vi "send_solutionChange-v01.vi"(0 "daq_ao 2":tag="Dev1/ao1", 1 "Duration (s)":dbl, 2 "controls array in":refnum<vi>[](array[refnum]), 3 "Sample Freq (Hz)":dbl min=0.0 max=40000.0, 4 "Phase":dbl, 5 "Duty Cycle":dbl, 6 "daq_ai":tag="Dev1/ai0:1", 8 "daq_do":tag="Dev1/ai0:1", 9 "Number of Replicates":i16=1 min=1 max=10, 10 "Start Position":T1(ring), 11 "common cluster":T2, 12 "Jump Position":T1(ring), 13 "error in":errorcluster) -> (14 "output cluster":T3={"daq_ao"="", "Duration (s)"=0.0, "Sample Freq (Hz)"=0.0, "Phase"=0.0, "Duty Cycle"=0.0, "Number of Replicates"=1} {"Number of Replicates" min=1 max=10}, 15 "output waveform":waveform(dbl), 16 "control array out":refnum<vi>[](array[refnum]), 18 "error out":errorcluster, 19 "jumptestMonitor":waveform(dbl)[](graph))   [LabVIEW 2019]
uses:
  multipatch/controls/multipatch_common_controls_v4.ctl
  machine_vision/controls/transform_cluster_actuator.ctl
  machine_vision/coordinate model vis/transform_properties_actuators.ctl
  pipette cleaning/pressure box/cleaning_soft/controls/actuator_cluster.ctl
  pipette cleaning/pressure box/cleaning_soft/controls/actuator_type.ctl
  pipette cleaning/pressure box/cleaning_soft/controls/pressure_box_control.ctl
  pipette cleaning/pressure box/cleaning_soft/controls/pressure_box_type.ctl
  controls/NH_method.ctl
  <vilib>/measure/NI_MABase.lvlib
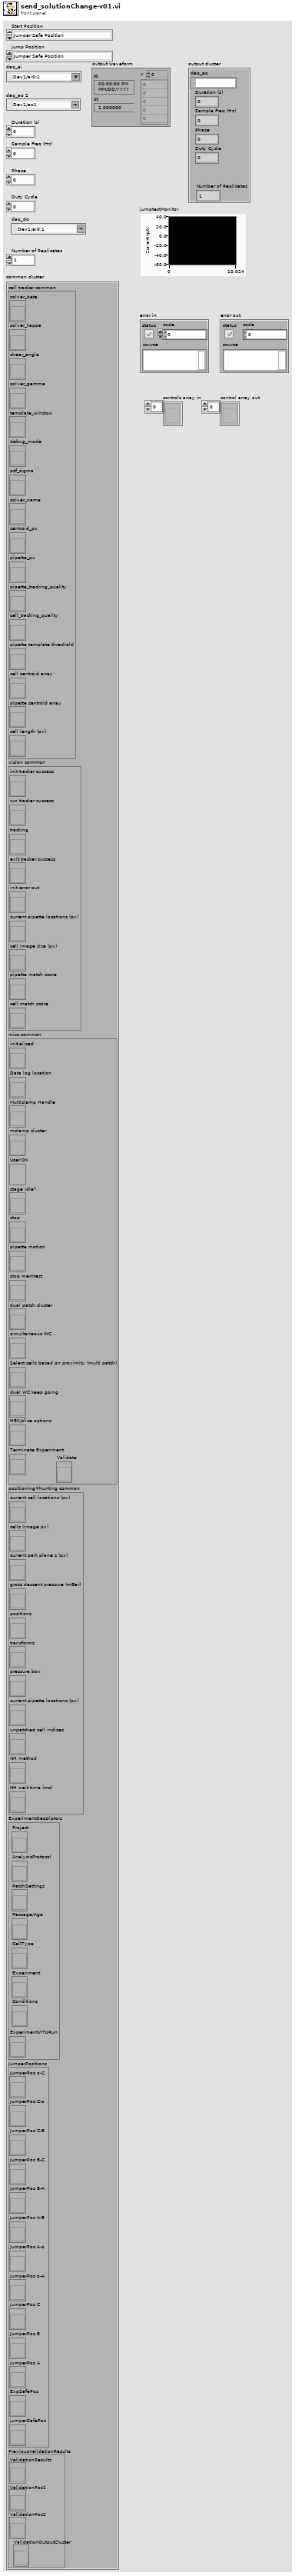
[diagram p1: front panel]
types:
  T1 = enum16{"Jumper Safe Position", "Experiment Safe Position", "Jumper Position A", "Jumper Position B", "Jumper Position C", "Jumper Position o-A", "Jumper Position A-o", "Jumper Position A-B", "Jumper Position B-A", "Jumper Position B-C", "Jumper Position C-B", "Jumper Position C-o", "Jumper Position o-C"}
  T2 = typedef "multipatch_common_controls_v4.ctl" = cluster{"cell tracker common":cluster{"solver_beta":refnum<vi>, "solver_kappa":refnum<vi>, "shear_angle":refnum<vi>, "solver_gamma":refnum<vi>, "template_window":refnum<vi>, "debug_mode":refnum<vi>, "psf_sigma":refnum<vi>, "solver_name":refnum<vi>, "centroid_px":refnum<vi>, "pipette_px":refnum<vi>, "pipette_tracking_quality":refnum<vi>, "cell_tracking_quality":refnum<vi>, "pipette template threshold":refnum<vi>, "cell centroid array":refnum<vi>, "pipette centroid array":refnum<vi>, "cell length (px)":refnum<vi>}, "vision common":cluster{"init tracker success":refnum<vi>, "run tracker success":refnum<vi>, "tracking":refnum<vi>, "exit tracker success":refnum<vi>, "init error out":refnum<vi>, "current pipette locations (px)":refnum<vi>, "cell image size (px)":refnum<vi>, "pipette match score":refnum<vi>, "cell match score":refnum<vi>}, "misc common":cluster{"initialized":refnum<vi>, "Data log location":refnum<vi>, "Multiclamp Handle":refnum<vi>, "mclamp cluster":refnum<vi>, "User OK":refnum<vi>, "stage idle?":refnum<vi>, "stop":refnum<vi>, "pipette motion":refnum<vi>, "stop memtest":refnum<vi>, "dual patch cluster":refnum<vi>, "simultaneous WC":refnum<vi>, "Select cells based on proximity (multi patch)":refnum<vi>, "dual WC keep going":refnum<vi>, "HEK/slice options":refnum<vi>, "Terminate Experiment":refnum<vi>, "Validate":refnum<vi>}, "positioning+hunting common":cluster{"current cell locations (px)":refnum<vi>, "cells (image px)":refnum<vi>, "current park plane z (px)":refnum<vi>, "gross descent pressure (mBar)":refnum<vi>, "positions":refnum<vi>, "transforms":refnum<vi>, "pressure box":refnum<vi>, "current pipette locations (px)":refnum<vi>, "unpatched cell indices":refnum<vi>, "NH method":refnum<vi>, "NH wait time (ms)":refnum<vi>}, "ExperimentDescriptors":cluster{"Project":refnum<vi>, "AnalysisProtocol":refnum<vi>, "PatchSettings":refnum<vi>, "Passage/Age":refnum<vi>, "CellType":refnum<vi>, "Experiment":refnum<vi>, "Conditions":refnum<vi>, "ExperimentVIToRun":refnum<vi>}, "JumperPositions":cluster{"JumperPos o-C":refnum<vi>, "JumperPos C-o":refnum<vi>, "JumperPos C-B":refnum<vi>, "JumperPos B-C":refnum<vi>, "JumperPos B-A":refnum<vi>, "JumperPos A-B":refnum<vi>, "JumperPos A-o":refnum<vi>, "JumperPos o-A":refnum<vi>, "JumperPos C":refnum<vi>, "JumperPos B":refnum<vi>, "JumperPos A":refnum<vi>, "ExpSafePos":refnum<vi>, "jumperSafePos":refnum<vi>}, "PreviousValidationResults":cluster{"ValidationResults":refnum<vi>, "ValidationPos1":refnum<vi>, "ValidationPos2":refnum<vi>, "ValidationOutputCluster":refnum<vi>}}
  T3 = cluster{"daq_ao":tag, "Duration (s)":dbl, "Sample Freq (Hz)":dbl, "Phase":dbl, "Duty Cycle":dbl, "Number of Replicates":i16}
  T4 = cluster{"daq_ao 2":tag, "Duration (s)":dbl, "Sample Freq (Hz)":dbl, "Phase":dbl, "Duty Cycle":dbl, "Number of Replicates":i16}
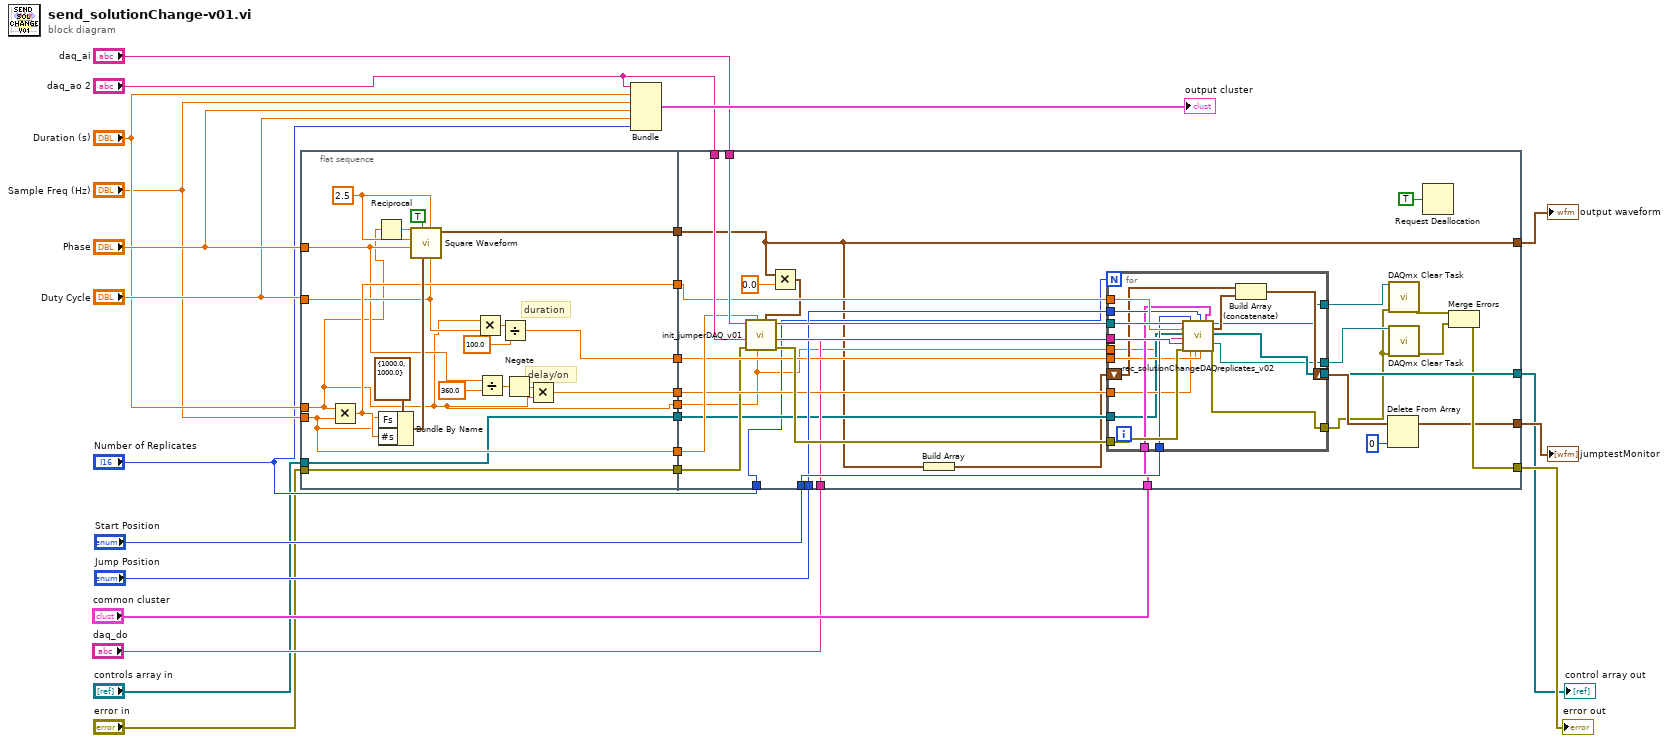
[diagram p0: block diagram]
diagram:
  n1 = flat-sequence {
    tunnel: "Phase" -> [w36]
    tunnel: "Duty Cycle" -> [w39]
    tunnel: "Duration (s)" -> [w27]
    tunnel: "Sample Freq (Hz)" -> [w41]
    tunnel: [w42] -> w17
    tunnel: [w41] -> w15
    tunnel: [w40] -> w16
    tunnel: [w32] -> w11
    tunnel: [w31] -> w10
    tunnel: "error in" -> [w29]
    tunnel: [w29] -> w6
    tunnel: "controls array in" -> [w28]
    tunnel: [w28] -> w4
    tunnel: [w27] -> w1
    tunnel: [w47] -> w22
    tunnel: w17 -> [w71]
    tunnel: w16 -> [w47]
    tunnel: "daq_ai" -> [w75]
    tunnel: "daq_ao 2" -> [w74]
    tunnel: w15 -> [w73]
    tunnel: [w51] -> w19
    tunnel: "Number of Replicates" -> [w59]
    tunnel: "Start Position" -> [w68]
    tunnel: "Jump Position" -> [w67]
    tunnel: "common cluster" -> [w66]
    tunnel: w11 -> [w65]
    tunnel: w10 -> [w64]
    tunnel: "daq_do" -> [w63]
    tunnel: w6 -> [w62]
    tunnel: [w54] -> w5
    tunnel: w4 -> [w61]
    tunnel: [w60] -> w3
    tunnel: w1 -> [w49]
    frame #0 {
      w46 = 2.5 ("Amplitude")
      # "delay/on"
      # "duration"
      n2 = Multiply(x=w27, y=w41) -> (x*y=w42:dbl)
      n3 = Reciprocal(x=w27) -> (1/x=w30:dbl)
      n4 = Bundle By Name(cluster=cluster{"Fs":dbl, "#s":dbl} {"Fs"=1000.0, "#s"=1000.0} ("sampling info"), "Fs"=w41, "#s"=w42) -> (w43:cluster{"Fs":dbl, "#s":dbl})
      n5 = call <vilib>:"Square Waveform.vi"("duty cycle (%)"=w39, "offset"=w46, "sampling info"=w43, "reset signal"=TRUE, "phase"=w36, "amplitude"=w46, "frequency"=w30) -> ("signal out"=w40:waveform(dbl))  [unwired: 3 in, 1 out]
      n6 = Multiply(x=w27, y=w39) -> (x*y=w38:dbl)
      n7 = Divide(x=w36, y=360.0) -> (x/y=w34:dbl)
      n8 = Divide(x=w38, y=100.0) -> (x/y=w32:dbl)
      n9 = Negate(x=w34) -> (-x=w33:dbl)
      n10 = Multiply(x=w33, y=w27) -> (x*y=w31:dbl)
    }
    frame #1 {
      n11 = Multiply(x=w47, y=0.0) -> (x*y=w69:waveform(dbl))
      n12 = call "init_jumperDAQ_v01.vi"("protocol waveform"=w69, "Duration (s)"=w49, "Sample Freq (Hz)"=w73, "AO error in"=w62, "AO physical channels"=w74, "AI Physical Channel"=w75) -> ("AO error out"=w78:errorcluster, "AO task out"=w77:refnum<k21>, "AI task out"=w76:refnum<k21>)  [unwired: 1 in, 2 out]
      n13 = Build Array(w47) -> (w52:waveform(dbl)[])
      n14 = for {
        N: w59 -> [_]
        tunnel: w77 -> [w96]
        tunnel: w76 -> [w95]
        tunnel: w71 -> [w93]
        tunnel: w68 -> [w92]
        tunnel: w67 -> [w91]
        tunnel: w66 -> [w90]
        tunnel: w65 -> [w89]
        tunnel: w64 -> [w88]
        tunnel: w63 -> [w87]
        tunnel: w61 -> [w86]
        tunnel: [w85] -> w60
        shift-right: [w83] -> w72
        shift-left: w52 -> [w82]
        tunnel: w78 -> [w97]
        tunnel: [w94] -> w56
        tunnel: [w81] -> w58
        tunnel: [w80] -> w57
        tunnel: w49 -> [w79]
        n15 = call "rec_solutionChangeDAQreplicates_v02.vi"("AI task in"=w95, "number of samples"=w93, "controls array in"=w86, "daq_do"=w87, "AO task in"=w96, "error in"=w97, "Start Position"=w92, "Jump On Time (s)"=w88, "Duration (s)"=w79, "Jump Position"=w91, "Jump Duration (s)"=w89, "common cluster"=w90) -> ("AI task out"=w81:refnum<k21>, "data out (pA or mV)"=w84:waveform(dbl), "control array out"=w85:refnum<vi>[], "AO task out"=w80:refnum<k21>, "error out"=w94:errorcluster)  [unwired: 3 in]
        n16 = Build Array (concatenate)(w82, w84) -> (w83:waveform(dbl)[])
      }
      n17 = Delete From Array(array=w72, index=0) -> (array with subset deleted=w51:waveform(dbl)[])  [unwired: 1 in, 1 out]
      n18 = call <vilib>:"DAQmx Clear Task.vi"("task in"=w58, "error in"=w56) -> ("error out"=w55:errorcluster)  [unwired: 13 in]
      n19 = call <vilib>:"DAQmx Clear Task.vi"("task in"=w57, "error in"=w56) -> ("error out"=w53:errorcluster)  [unwired: 13 in]
      n20 = Request Deallocation(TRUE ("flag")) -> ()
      n21 = Merge Errors(w55, w53) -> (w54:errorcluster)
    }
  }
  n22 = Bundle("daq_ao 2"="daq_ao 2", "Duration (s)"="Duration (s)", "Sample Freq (Hz)"="Sample Freq (Hz)", "Phase"="Phase", "Duty Cycle"="Duty Cycle", "Number of Replicates"="Number of Replicates") -> (→"output cluster":T4)  [unwired: 1 in]
  "jumptestMonitor" <- w19
  "output waveform" <- w22
  "error out" <- w5
  "control array out" <- w3
